vi "sequence filter.vi"(0 "seq in":string[][](array[string])=[["0", "", "100"], ["1", "", "1"], ["2", "", "1"], ["3", "", "1"], ["4", "", "1"], ["5", "", "1"], ["6", "", "1"], ["7", "", "1"], ["8", "", "100"]], 3 "Magnet":T1) -> (2 "seq  out":string[][](array[string]))   [LabVIEW 2021]
uses:
  Ctl/magnet.ctl
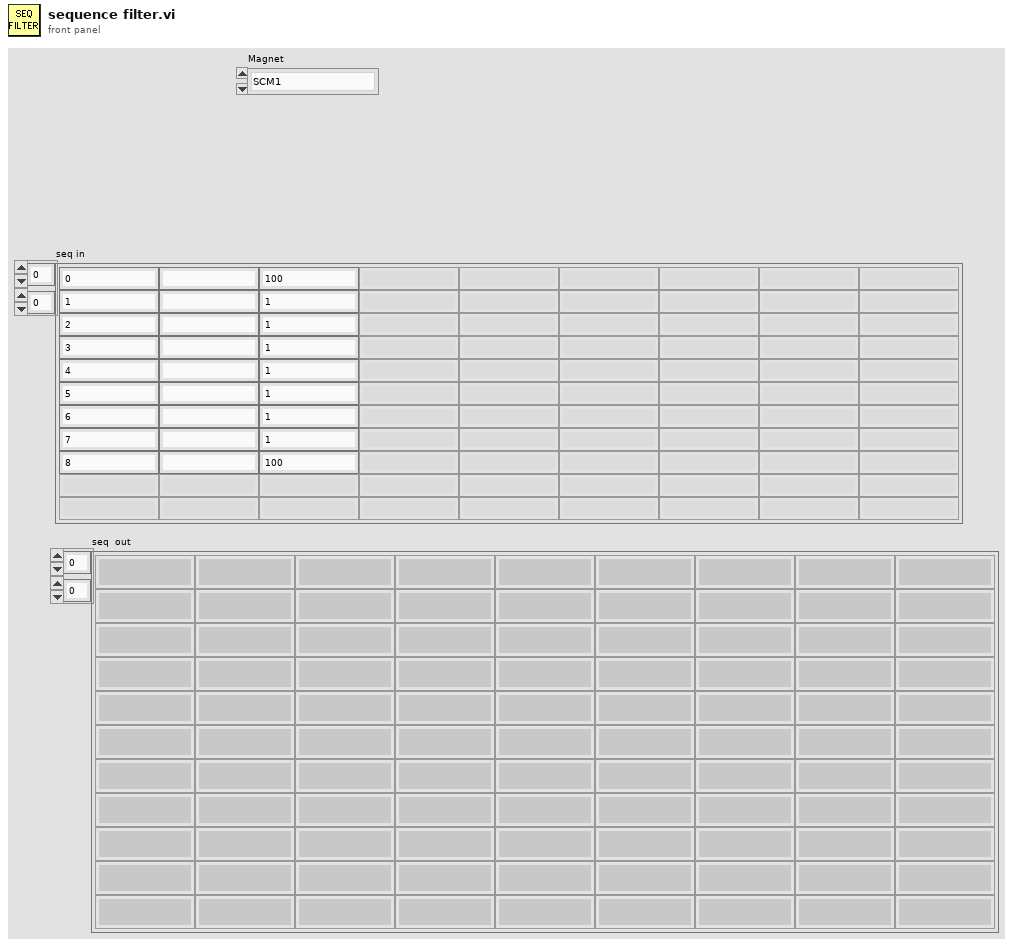
[diagram p1: front panel]
types:
  T1 = typedef "magnet.ctl" = enum16{"SCM1", "SCM2", "SCM3", "SCMX", "Cell8", "Cell9", "Cell12", "Hybrid", "Great Magnet"}
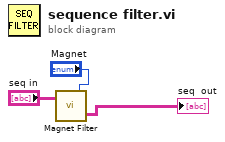
[diagram p0: block diagram]
diagram:
  n1 = call "Magnet Filter.vi"("Magnet"="Magnet", "seq in"="seq in") -> ("seq  out"=→"seq  out":string[][])  [unwired: 1 in]
